vi "FTW-Logger-NewLogFile.vi"(0 "FTW Logger":refnum<class "FTW-Logger-Core.lvclass">, 11 "error in":errorcluster) -> (4 "FTW Logger out":refnum<class "FTW-Logger-Core.lvclass">, 15 "error out":errorcluster)   [LabVIEW 2013, in "FTW-Logger-Core.lvclass"]
uses:
  FTW-Logger-Core.lvclass
  Time/FTW-Time-DisplayFormat-Timestamp.ctl
  FTW-Logger-Core.lvclass/FTW-Logger-Core.ctl
panel:
  # "Inputs"
  # "Outputs"
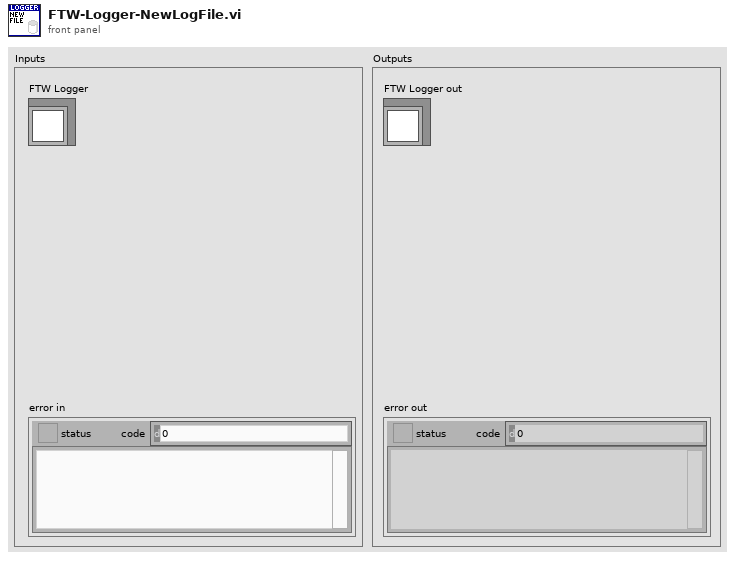
[diagram p1: front panel]
types:
  T1 = typedef "FTW-Time-DisplayFormat-Timestamp.ctl" = enum16{"YYYY-MM-DDT00:00:00.000Z (UTC)", "YYYY-MM-DDT00:00:00.000 (locale)", "YYYY-MM-DDT00:00:00.000+hh:mm (time zone)", "YYYY-MM-DDT00-00-00Z (simple UTC)", "YYYY-MM-DDT00-00-00 (simple locale)", "YYYY-MM-DD"}
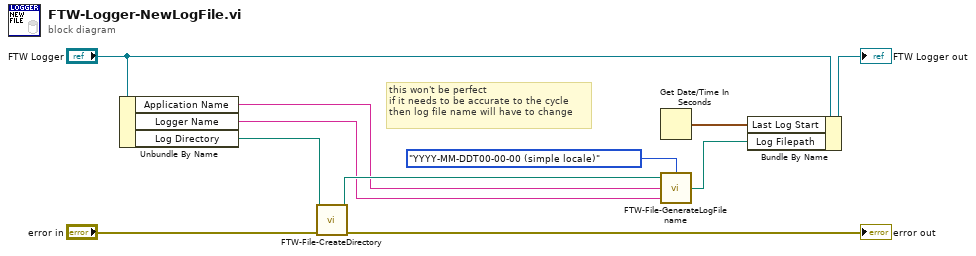
[diagram p0: block diagram]
diagram:
  # "this won't be perfect\nif it needs to be accurate to the cycle\nthen log file name will have to change"
  n1 = Unbundle By Name("FTW Logger") -> ("Application Name"=w7:string, "Logger Name"=w6:string, "Log Directory"=w9:path)
  n2 = call "FTW-File-CreateDirectory.vi"("Directory to Create"=w9, "error in"="error in") -> ("Created Directory"=w10:path, "error out"=→"error out":errorcluster)  [unwired: 12 in]
  n3 = Get Date/Time In Seconds() -> (seconds since 1Jan1904=w5:timestamp)
  n4 = call "FTW-File-GenerateLogFilename.vi"("Date Format"=FTW-Time-DisplayFormat-Timestamp."YYYY-MM-DDT00-00-00 (simple locale)", "Type"=w6, "Application"=w7, "Directory"=w10) -> ("Filepath"=w8:path)
  n5 = Bundle By Name(cluster="FTW Logger", "Last Log Start"=w5, "Log Filepath"=w8) -> (→"FTW Logger out":refnum<class "FTW-Logger-Core.lvclass">)
